vi "RT_DynamicPressure.vi"(8 "V (m/s)":dbl[](array[numeric]), 10 "V_wind (m/s)":dbl[](array[numeric]), 11 "h (m)":dbl format="%#_13g") -> (0 "Patm (Pa)":dbl, 3 "Pdin":dbl)   [LabVIEW 2017]
uses:
  <vilib>/Analysis/_algsub.llb/Vector Norm Type.ctl
  <vilib>/Analysis/_algsub.llb/Real Vector Norm.vi
  <vilib>/Analysis/NI_AALPro.lvlib
panel:
  out "rho (kg/m^3)":dbl
  out "p (Pa)":dbl
  out "T(ºC)":dbl
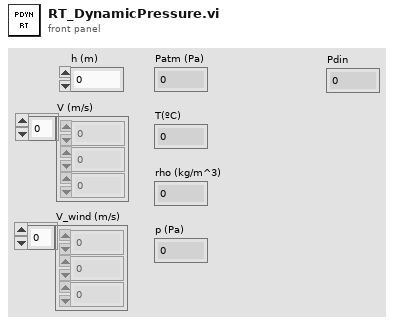
[diagram p1: front panel]
types:
  T1 = typedef "NI_AALPro.lvlib/Vector Norm Type.ctl" = u16
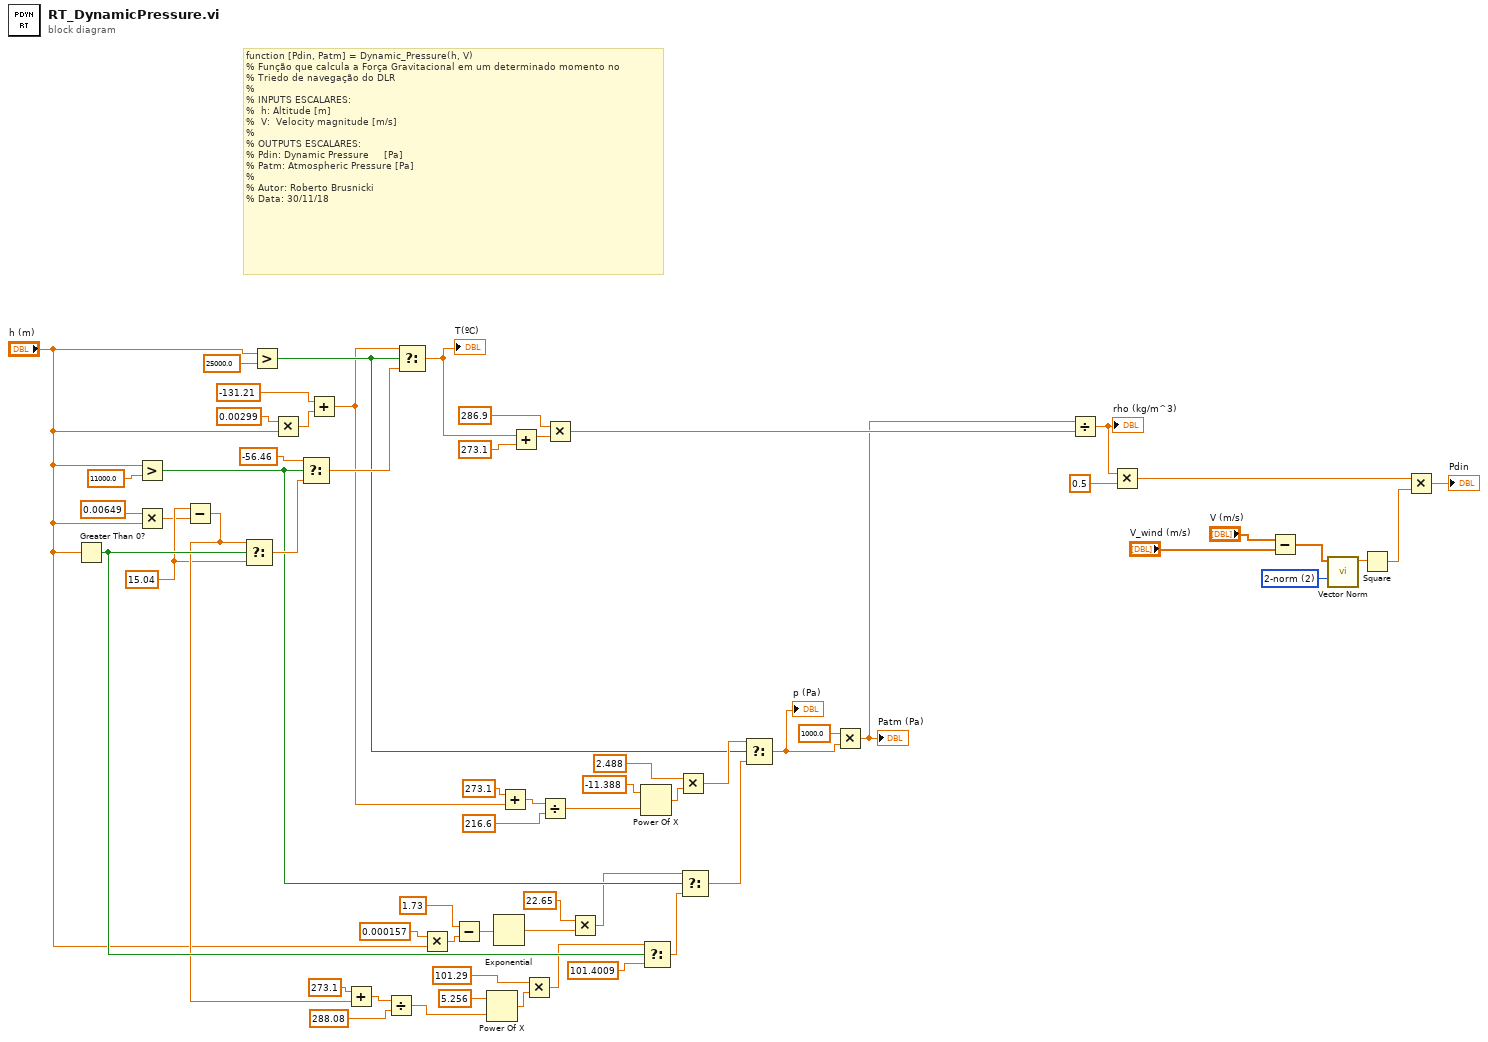
[diagram p0: block diagram]
diagram:
  w11 = T1 2 items=["1-norm"=1, "2-norm"=2, "Inf-norm"=3, "-Inf-norm"=4, "User Defined"=5] ("norm type")
  w39 = 15.04 ("x")
  # "function [Pdin, Patm] = Dynamic_Pressure(h, V)\n% Função que calcula a Força Gravitacional em um determinado momento no \n% Triedo de navegação do DLR\n%\n% INPUTS ESCALARES:\n%  h: Altitude [m]\n%  V:  Velocity magnitude [m/s]\n%\n% OUTPUTS ESCALARES:\n% Pdin: Dynamic Pressure     [Pa]\n% Patm: Atmospheric Pressure [Pa]\n%\n% Autor: Roberto Brusnicki\n% Data: 30/11/18"
  n1 = Greater Than 0?(x="h (m)") -> (x > 0?=w48:bool)
  n2 = Greater?(x="h (m)", y=11000.0) -> (0:w33:bool)
  n3 = Multiply(x=0.00649 ("y"), y="h (m)") -> (x*y=w35:dbl)
  n4 = Subtract(x=w39, y=w35) -> (x-y=w46:dbl)
  n5 = Select(t=w46, s=w48, f=w39) -> (s? t:f=w38:dbl)
  n6 = Greater?(x="h (m)", y=25000.0) -> (0:w16:bool)
  n7 = Multiply(x=0.00299 ("y"), y="h (m)") -> (x*y=w14:dbl)
  n8 = Select(t=-56.46, s=w33, f=w38) -> (s? t:f=w24:dbl)
  n9 = Add(x=-131.21 ("y"), y=w14) -> (x+y=w1:dbl)
  n10 = Add(x=273.1 ("y"), y=w46) -> (x+y=w44:dbl)
  n11 = Divide(x=w44, y=288.08) -> (x/y=w6:dbl)
  n12 = Select(t=w1, s=w16, f=w24) -> (s? t:f=w2:dbl)
  "T(ºC)" <- w2
  n13 = Multiply(x=0.000157 ("y"), y="h (m)") -> (x*y=w27:dbl)
  n14 = Subtract(x=1.73, y=w27) -> (x-y=w29:dbl)
  n15 = Power Of X(1:w6, 2:5.256 ("x")) -> (0:w41:dbl)
  n16 = Exponential(1:w29) -> (0:w30:dbl)
  n17 = Add(x=273.1 ("y"), y=w1) -> (x+y=w18:dbl)
  n18 = Add(x=w2, y=273.1) -> (x+y=w53:dbl)
  n19 = Multiply(x=101.29, y=w41) -> (x*y=w47:dbl)
  n20 = Divide(x=w18, y=216.6) -> (x/y=w8:dbl)
  n21 = Multiply(x=286.9, y=w53) -> (x*y=w56:dbl)
  n22 = Multiply(x=22.65, y=w30) -> (x*y=w32:dbl)
  n23 = Power Of X(1:w8, 2:-11.388 ("x")) -> (0:w25:dbl)
  n24 = Select(t=w47, s=w48, f=101.4009) -> (s? t:f=w40:dbl)
  n25 = Multiply(x=2.488, y=w25) -> (x*y=w21:dbl)
  n26 = Select(t=w32, s=w33, f=w40) -> (s? t:f=w34:dbl)
  n27 = Select(t=w21, s=w16, f=w34) -> (s? t:f=w50:dbl)
  "p (Pa)" <- w50
  n28 = Multiply(x=1000.0, y=w50) -> (x*y=w55:dbl)
  "Patm (Pa)" <- w55
  n29 = Divide(x=w55, y=w56) -> (x/y=w58:dbl)
  "rho (kg/m^3)" <- w58
  n30 = Multiply(x=w58, y=0.5 ("x")) -> (x*y=w59:dbl)
  n31 = Subtract(x="V (m/s)", y="V_wind (m/s)") -> (x-y=w3:dbl[])
  n32 = call-poly <vilib>:"Vector Norm.vi"("norm type"=w11, "Input Vector"=w3) -> ("norm"=w10:dbl)  [unwired: 8 in, 1 out]
  n33 = Square(x=w10) -> (x^2=w60:dbl)
  n34 = Multiply(x=w59, y=w60) -> (x*y=→"Pdin":dbl)
